vi "keccak.ip.ctrl.vi"(11 "Reset":bool) -> ()   [LabVIEW 2021]
uses:
  Users/johns/OneDrive/Documents/LabVIEW Data/Untitled Project 2/CLIP/keccak.variables.ctl
  Users/johns/OneDrive/Documents/LabVIEW Data/Untitled Project 2/CLIP/keccak.states.ctl
panel:
  in  "State.in":T1={"hash.input_size"=0, "hash.bits"=0, "state.next"=enum."Wait.for.Start", "state.after_next"=enum."Wait.for.Start", "read.i"=0, "read.block_i"=0, "hash.block_words"=0, "hash.block_size"=0, "keccak.i"=0, "state[25]"=[0, 0, 0, 0, 0, 0, 0, 0, 0, 0, 0, 0, 0, 0, 0, 0, 0, 0, 0, 0, 0, 0, 0, 0, 0], "HT_PARMS.Valid"=FALSE, "HT_PARMS.Data"=0, "Read.HT_PARMS"=FALSE, "HT_DATA.Valid"=FALSE, "HT_DATA.Data"=0, "Read.HT_DATA"=FALSE, "TH_RESULTS.Valid"=FALSE, "TH_RESULTS.Data"=0, "TH_RESULTS.Ready"=FALSE}
  out "State.Out":T1={"hash.input_size"=0, "hash.bits"=0, "state.next"=enum."Wait.for.Start", "state.after_next"=enum."Wait.for.Start", "read.i"=0, "read.block_i"=0, "hash.block_words"=0, "hash.block_size"=0, "keccak.i"=0, "state[25]"=[0, 0, 0, 0, 0, 0, 0, 0, 0, 0, 0, 0, 0, 0, 0, 0, 0, 0, 0, 0, 0, 0, 0, 0, 0], "HT_PARMS.Valid"=FALSE, "HT_PARMS.Data"=0, "Read.HT_PARMS"=FALSE, "HT_DATA.Valid"=FALSE, "HT_DATA.Data"=0, "Read.HT_DATA"=FALSE, "TH_RESULTS.Valid"=FALSE, "TH_RESULTS.Data"=0, "TH_RESULTS.Ready"=FALSE}
  in  "HT_DATA.Valid":bool
  in  "HT_DATA.Data":u64
  in  "HT_PARMS.Valid":bool
  in  "HT_PARMS.Data":u64
  in  "TH_RESULTS.Ready":bool
  out "Read.HT_DATA":bool
  out "Read.HT_PARMS":bool
  out "TH_RESULTS.Valid":bool
  out "TH_RESULTS.Data":u64
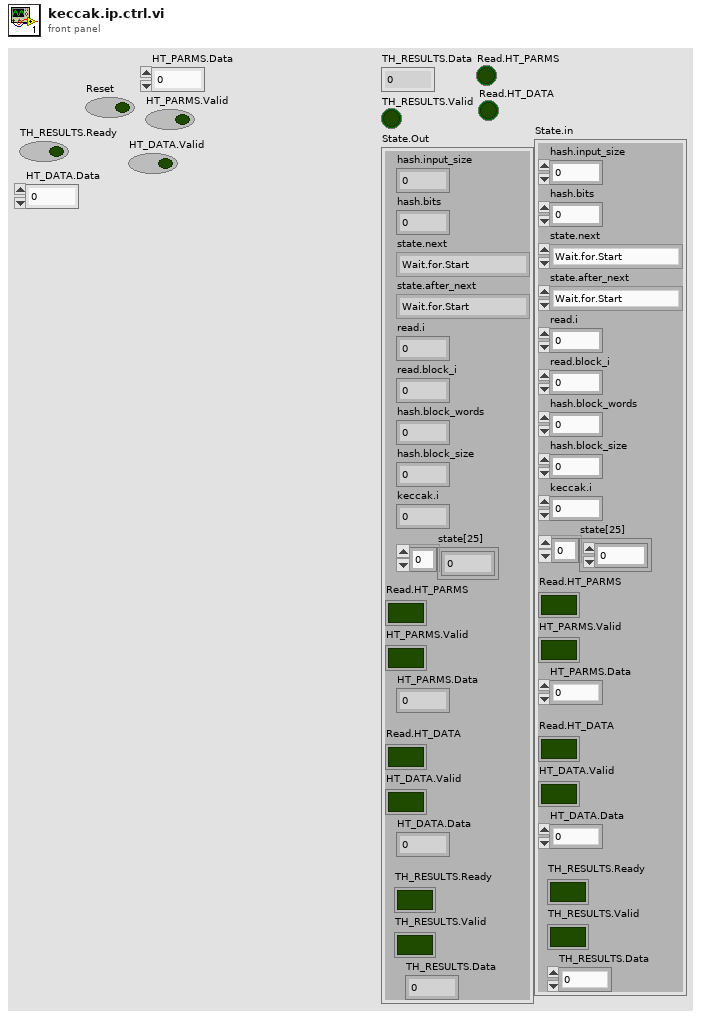
[diagram p1: front panel]
types:
  T1 = typedef "keccak.variables.ctl" = cluster{"hash.input_size":u16, "hash.bits":u16, "state.next":T2, "state.after_next":T2, "read.i":u16, "read.block_i":u16, "hash.block_words":u16, "hash.block_size":u16, "keccak.i":u16, "state[25]":u64[], "HT_PARMS.Valid":bool, "HT_PARMS.Data":u64, "Read.HT_PARMS":bool, "HT_DATA.Valid":bool, "HT_DATA.Data":u64, "Read.HT_DATA":bool, "TH_RESULTS.Valid":bool, "TH_RESULTS.Data":u64, "TH_RESULTS.Ready":bool}
  T2 = typedef "keccak.states.ctl" = enum8{"Wait.for.Start", "Read.Blocks", "Read.Remainder", "Keccak", "Send.Result"}
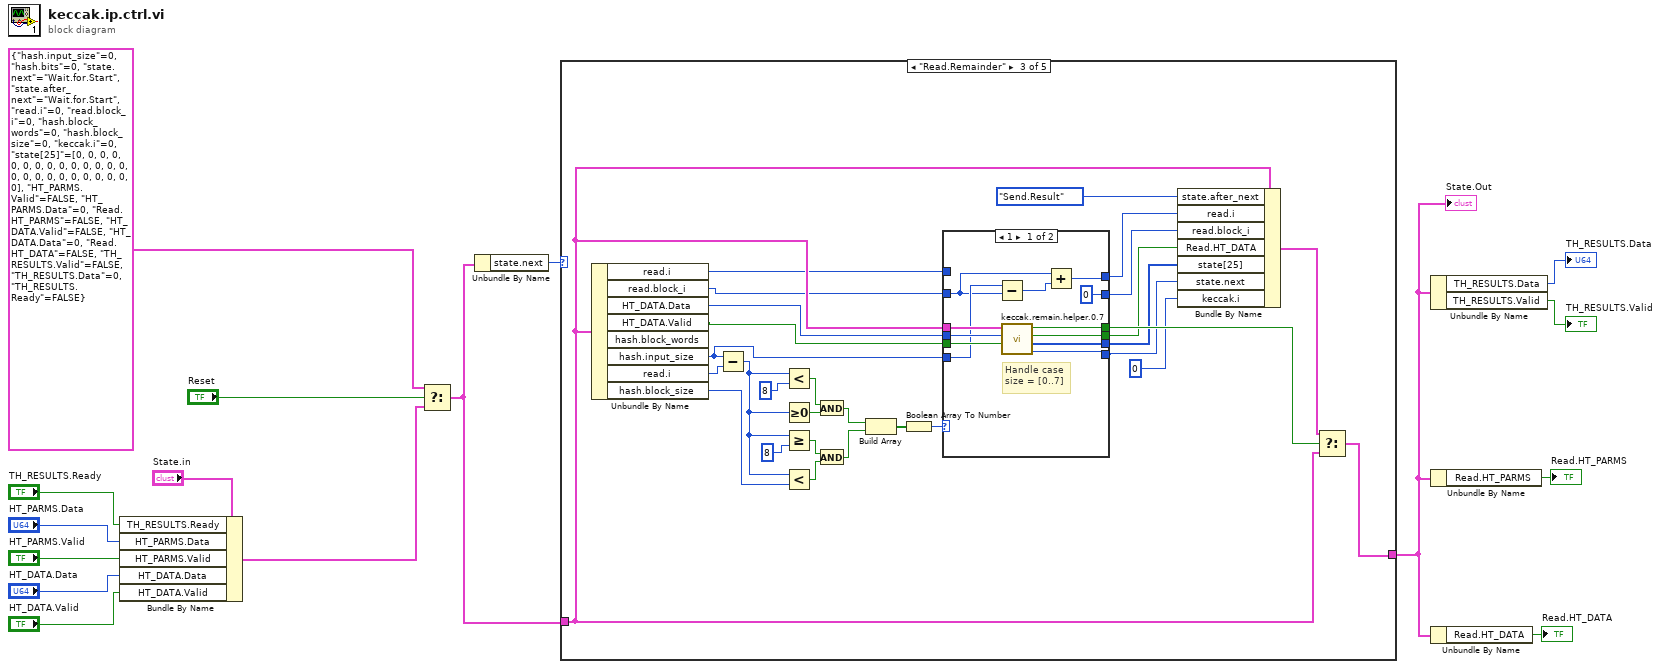
[diagram p0: block diagram]
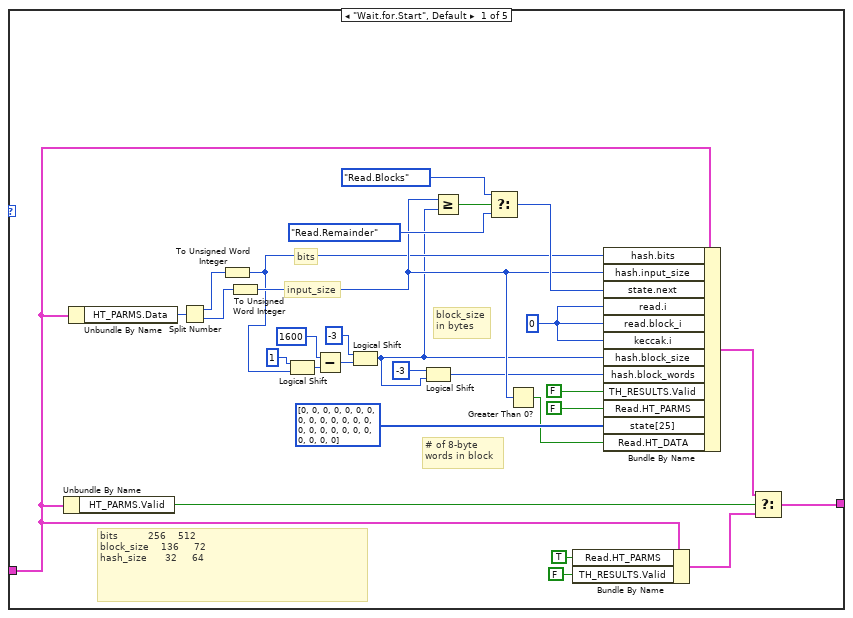
[diagram p2: hidden frame]
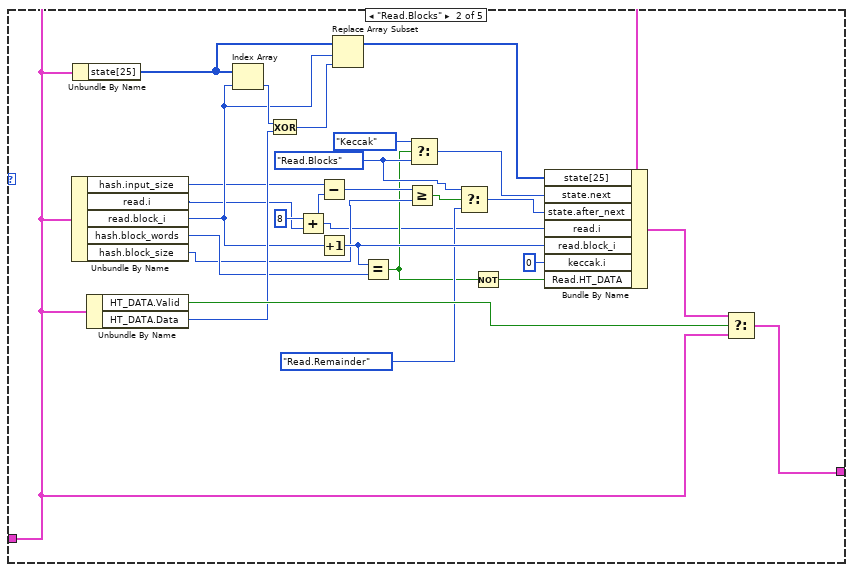
[diagram p3: hidden frame]
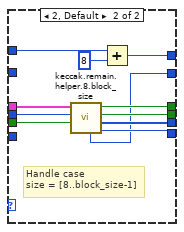
[diagram p4: hidden frame]
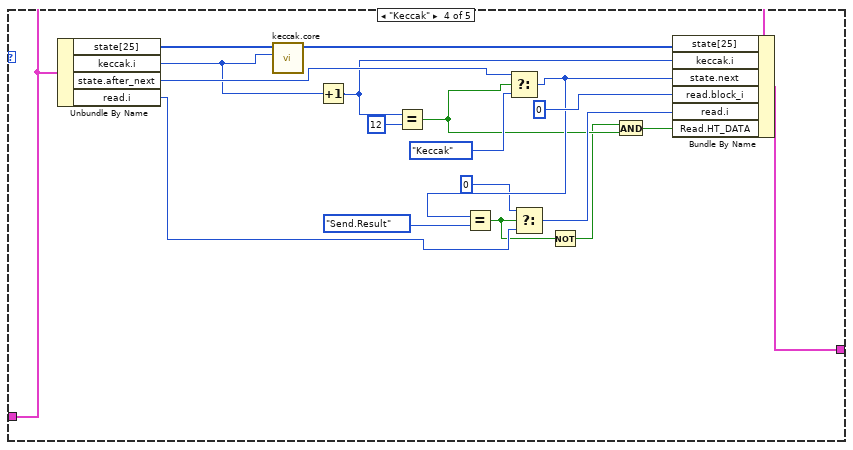
[diagram p5: hidden frame]
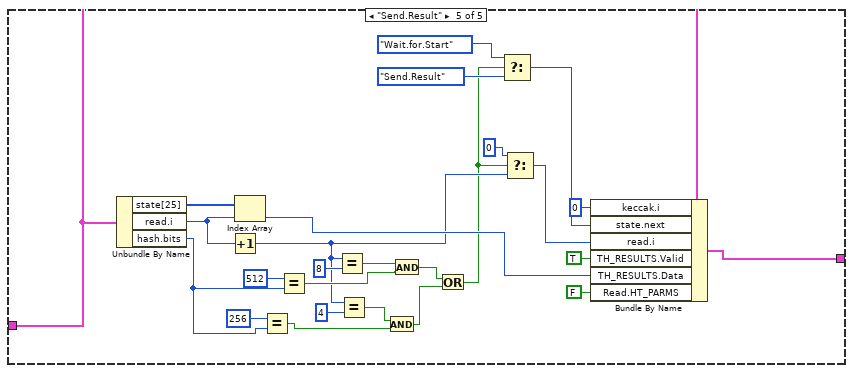
[diagram p6: hidden frame]
diagram:
  n1 = Bundle By Name(cluster="State.in", "TH_RESULTS.Ready"="TH_RESULTS.Ready", "HT_PARMS.Data"="HT_PARMS.Data", "HT_PARMS.Valid"="HT_PARMS.Valid", "HT_DATA.Data"="HT_DATA.Data", "HT_DATA.Valid"="HT_DATA.Valid") -> (w1:T1)
  n2 = Select(t=T1 {"hash.input_size"=0, "hash.bits"=0, "state.next"=enum."Wait.for.Start", "state.after_next"=enum."Wait.for.Start", "read.i"=0, "read.block_i"=0, "hash.block_words"=0, "hash.block_size"=0, "keccak.i"=0, "state[25]"=[0, 0, 0, 0, 0, 0, 0, 0, 0, 0, 0, 0, 0, 0, 0, 0, 0, 0, 0, 0, 0, 0, 0, 0, 0], "HT_PARMS.Valid"=FALSE, "HT_PARMS.Data"=0, "Read.HT_PARMS"=FALSE, "HT_DATA.Valid"=FALSE, "HT_DATA.Data"=0, "Read.HT_DATA"=FALSE, "TH_RESULTS.Valid"=FALSE, "TH_RESULTS.Data"=0, "TH_RESULTS.Ready"=FALSE} ("Variables"), s="Reset", f=w1) -> (s? t:f=w12:T1)
  n3 = Unbundle By Name(w12) -> ("state.next"=w16:T2)
  n4 = case shown="\"Read.Remainder\"" w16 {
    tunnel: [w41 w71 w98 w141 w169] -> w15
    tunnel: w12 -> [w36 w70 w94 w142 w168]
    frame "Wait.for.Start", Default {
      w26 = u16 0 ("read.i")
      # "# of 8-byte\nwords in block"
      # "block_size\nin bytes"
      # "bits"
      # "input_size"
      # "bits          256    512\nblock_size    136     72\nhash_size      32     64"
      n5 = Unbundle By Name(w36) -> ("HT_PARMS.Valid"=w40:bool)
      n6 = Unbundle By Name(w36) -> ("HT_PARMS.Data"=w45:u64)
      n7 = Split Number(x=w45) -> (hi(x)=w44:u32, lo(x)=w43:u32)
      n8 = To Unsigned Word Integer(number=w44) -> (unsigned 16bit integer=w18:u16)
      n9 = To Unsigned Word Integer(number=w43) -> (unsigned 16bit integer=w28:u16)
      n10 = Logical Shift(y=i16 1, x=w18) -> (x << y=w23:u16)
      n11 = Subtract(x=u16 1600, y=w23) -> (x-y=w22:u16)
      n12 = Logical Shift(y=i16 -3, x=w22) -> (x << y=w17:u16)
      n13 = Logical Shift(y=i16 -3, x=w17) -> (x << y=w19:u16)
      n14 = Greater Or Equal?(x=w28, y=w17) -> (x >= y?=w32:bool)
      n15 = Select(t=keccak.states."Read.Blocks" ("state.next"), s=w32, f=keccak.states."Read.Remainder" ("state.next")) -> (s? t:f=w30:T2)
      n16 = Greater Than 0?(x=w28) -> (x > 0?=w27:bool)
      n17 = Bundle By Name(cluster=w36, "Read.HT_PARMS"=TRUE, "TH_RESULTS.Valid"=FALSE) -> (w37:T1)
      n18 = Bundle By Name(cluster=w36, "hash.bits"=w18, "hash.input_size"=w28, "state.next"=w30, "read.i"=w26, "read.block_i"=w26, "keccak.i"=w26, "hash.block_size"=w17, "hash.block_words"=w19, "TH_RESULTS.Valid"=FALSE, "Read.HT_PARMS"=FALSE, "state[25]"=u64[] [0, 0, 0, 0, 0, 0, 0, 0, 0, 0, 0, 0, 0, 0, 0, 0, 0, 0, 0, 0, 0, 0, 0, 0, 0] ("state[24]"), "Read.HT_DATA"=w27) -> (w42:T1)
      n19 = Select(t=w42, s=w40, f=w37) -> (s? t:f=w41:T1)
    }
    frame "Read.Blocks" {
      w51 = keccak.states."Read.Blocks" ("state.next")
      n20 = Unbundle By Name(w70) -> ("hash.input_size"=w56:u16, "read.i"=w55:u16, "read.block_i"=w64:u16, "hash.block_words"=w60:u16, "hash.block_size"=w52:u16)
      n21 = Unbundle By Name(w70) -> ("state[25]"=w68:u64[])
      n22 = Unbundle By Name(w70) -> ("HT_DATA.Valid"=w69:bool, "HT_DATA.Data"=w65:u64)
      n23 = Index Array(array=w68, index=w64) -> (element=w67:u64)
      n24 = Exclusive Or(1:w65, 2:w67) -> (0:w66:u64)
      n25 = Add(x=u16 8, y=w55) -> (x+y=w46:u16)
      n26 = Subtract(x=w56, y=w46) -> (x-y=w53:u16)
      n27 = Increment(x=w64) -> (x+1=w61:u16)
      n28 = Replace Array Subset(array=w68, new element=w66, index=w64) -> (w57:u64[])
      n29 = Equal?(x=w61, y=w60) -> (x = y?=w48:bool)
      n30 = Greater Or Equal?(x=w53, y=w52) -> (x >= y?=w54:bool)
      n31 = Select(t=keccak.states."Keccak" ("state.next"), s=w48, f=w51) -> (s? t:f=w62:T2)
      n32 = Select(t=w51, s=w54, f=keccak.states."Read.Remainder" ("state.next")) -> (s? t:f=w58:T2)
      n33 = Not(x=w48) -> (.not. x?=w47:bool)
      n34 = Bundle By Name(cluster=w70, "state[25]"=w57, "state.next"=w62, "state.after_next"=w58, "read.i"=w46, "read.block_i"=w61, "keccak.i"=u16 0, "Read.HT_DATA"=w47) -> (w72:T1)
      n35 = Select(t=w72, s=w69, f=w70) -> (s? t:f=w71:T1)
    }
    frame "Read.Remainder" {
      n36 = Unbundle By Name(w94) -> ("read.i"=w78:u16, "read.block_i"=w79:u16, "HT_DATA.Data"=w93:u64, "HT_DATA.Valid"=w92:bool, "hash.input_size"=w77:u16, "read.i"=w101:u16, "hash.block_size"=w81:u16)  [unwired: 1 out]
      n37 = Subtract(x=w77, y=w101) -> (x-y=w82:u16)
      n38 = Less?(x=w82, y=u16 8) -> (x < y?=w90:bool)
      n39 = Greater Or Equal To 0?(x=w82) -> (x >= 0?=w91:bool)
      n40 = Greater Or Equal?(x=w82, y=u16 8) -> (x >= y?=w85:bool)
      n41 = Less?(x=w82, y=w81) -> (x < y?=w80:bool)
      n42 = And(x=w90, y=w91) -> (x .and. y?=w87:bool)
      n43 = And(x=w85, y=w80) -> (x .and. y?=w84:bool)
      n44 = Build Array(w87, w84) -> (w88:bool[])
      n45 = Boolean Array To Number(Boolean array=w88) -> (number=w86:u8)
      n46 = case shown="1" w86 {
        tunnel: [w113 w120] -> w97
        tunnel: [w112 w121] -> w96
        tunnel: [w111 w119] -> w95
        tunnel: w94 -> [w110 w124]
        tunnel: w93 -> [w109 w123]
        tunnel: w92 -> [w108 w122]
        tunnel: [w107 w115] -> w76
        tunnel: w79 -> [w104 _]
        tunnel: [u16 0 w114] -> w74
        tunnel: [w103 w117] -> w73
        tunnel: w78 -> [_ w116]
        tunnel: w77 -> [w105 _]
        frame 1 {
          # "Handle case\nsize = [0..7]"
          n47 = Subtract(x=w105, y=w104) -> (x-y=w102:u16)
          n48 = call "keccak.remain.helper.0.7.vi"("HT_DATA.Valid"=w108, "HT_DATA.Data"=w109, "Variables"=w110) -> ("state.next"=w107:T2, "state[25] out"=w111:u64[], "Continue?"=w112:bool, "Valid"=w113:bool)  [unwired: 5 in]
          n49 = Add(x=w104, y=w102) -> (x+y=w103:u16)
        }
        frame 2, Default {
          # "Handle case\nsize = [8..block_size-1]"
          n50 = call "keccak.remain.helper.8.block_size.vi"("HT_DATA.Valid"=w122, "HT_DATA.Data"=w123, "Variables"=w124) -> ("state.next"=w115:T2, "state[25] out"=w119:u64[], "Continue?"=w121:bool, "Valid"=w120:bool, "read.block_i"=w114:u16)  [unwired: 4 in]
          n51 = Add(x=w116, y=u16 8) -> (x+y=w117:u16)
        }
      }
      n52 = Bundle By Name(cluster=w94, "state.after_next"=keccak.states."Send.Result" ("state.next"), "read.i"=w73, "read.block_i"=w74, "Read.HT_DATA"=w96, "state[25]"=w95, "state.next"=w76, "keccak.i"=u16 0) -> (w99:T1)
      n53 = Select(t=w99, s=w97, f=w94) -> (s? t:f=w98:T1)
    }
    frame "Keccak" {
      n54 = Unbundle By Name(w142) -> ("state[25]"=w143:u64[], "keccak.i"=w135:u16, "state.after_next"=w137:T2, "read.i"=w132:u16)
      n55 = call "keccak.core.vi"("keccak.i"=w135, "state[25]"=w143) -> ("state[25].out"=w140:u64[])  [unwired: 9 in]
      n56 = Increment(x=w135) -> (x+1=w136:u16)
      n57 = Equal?(x=w136, y=u16 12) -> (x = y?=w128:bool)
      n58 = Select(t=w137, s=w128, f=keccak.states."Keccak" ("state.next")) -> (s? t:f=w131:T2)
      n59 = Equal?(x=w131, y=keccak.states."Send.Result" ("state.next")) -> (x = y?=w126:bool)
      n60 = Select(t=u16 0, s=w126, f=w132) -> (s? t:f=w133:u16)
      n61 = Not(x=w126) -> (.not. x?=w125:bool)
      n62 = And(x=w125, y=w128) -> (x .and. y?=w127:bool)
      n63 = Bundle By Name(cluster=w142, "state[25]"=w140, "keccak.i"=w136, "state.next"=w131, "read.block_i"=u16 0 ("read.i"), "read.i"=w133, "Read.HT_DATA"=w127) -> (w141:T1)
    }
    frame "Send.Result" {
      n64 = Unbundle By Name(w168) -> ("state[25]"=w167:u64[], "read.i"=w166:u16, "hash.bits"=w156:u16)
      n65 = Increment(x=w166) -> (x+1=w149:u16)
      n66 = Index Array(array=w167, index=w166) -> (element=w157:u64)
      n67 = Equal?(x=u16 256, y=w156) -> (x = y?=w153:bool)
      n68 = Equal?(x=u16 512, y=w156) -> (x = y?=w162:bool)
      n69 = Equal?(x=w149, y=u16 8) -> (x = y?=w163:bool)
      n70 = Equal?(x=w149, y=u16 4) -> (x = y?=w152:bool)
      n71 = And(x=w152, y=w153) -> (x .and. y?=w151:bool)
      n72 = And(x=w163, y=w162) -> (x .and. y?=w150:bool)
      n73 = Or(x=w150, y=w151) -> (x .or. y?=w147:bool)
      n74 = Select(t=keccak.states."Wait.for.Start" ("state.next"), s=w147, f=keccak.states."Send.Result" ("state.next")) -> (s? t:f=w159:T2)
      n75 = Select(t=u16 0, s=w147, f=w149) -> (s? t:f=w148:u16)
      n76 = Bundle By Name(cluster=w168, "keccak.i"=u16 0, "state.next"=w159, "read.i"=w148, "TH_RESULTS.Valid"=TRUE, "TH_RESULTS.Data"=w157, "Read.HT_PARMS"=FALSE) -> (w169:T1)
    }
  }
  "State.Out" <- w15
  n77 = Unbundle By Name(w15) -> ("TH_RESULTS.Data"=→"TH_RESULTS.Data":u64, "TH_RESULTS.Valid"=→"TH_RESULTS.Valid":bool)
  n78 = Unbundle By Name(w15) -> ("Read.HT_PARMS"=→"Read.HT_PARMS":bool)
  n79 = Unbundle By Name(w15) -> ("Read.HT_DATA"=→"Read.HT_DATA":bool)
